vi "Disconnect.vi"(6 "Timeout ms (1000)":i32=1000, 8 "error in (no error)":errorcluster, 11 "NetworkConnection in":refnum<class "NetworkConnection.lvclass">) -> (0 "error out":errorcluster, 3 "NetworkConnection out":refnum<class "NetworkConnection.lvclass">)   [LabVIEW 2020, in "NetworkConnection.lvclass"]
doc: "Disconnects the Network Connection. All unread messages will be flushed.\nJKI Network Streams Connection 1.1.1.15\nJavier Ruiz - JKI\nCopyright (c) 2020, JKI\n\nThis library is provided \"AS IS\" ,WITHOUT WARRANTIES OR CONDITIONS OF ANY KIND, either express or implied."
uses:
  NetworkConnection.lvclass
  Flush And Wait Empty Condition.ctl
  NetworkMessage--Cluster.ctl
  NetworkCommand--Cluster.ctl
  NetworkConnection.lvclass/NetworkConnection.ctl
panel:
  # "Copyright © 2020 JKI All rights reserved.\n\nAuthor: Javier Ruiz <javier.ruiz@jki.net>\n\nThis library is provided \"AS IS\" ,WITHOUT WARRANTIES OR \nCONDITIONS OF ANY KIND, either expressed or implied.\n\nJKI -- jki.net"
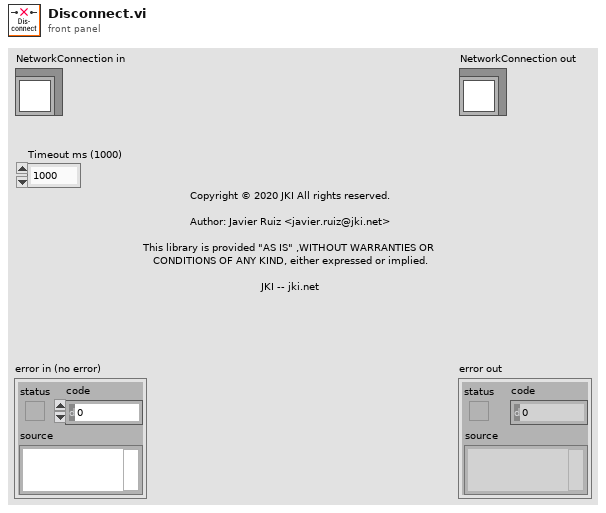
[diagram p1: front panel]
types:
  T1 = typedef "Flush And Wait Empty Condition.ctl" = u8
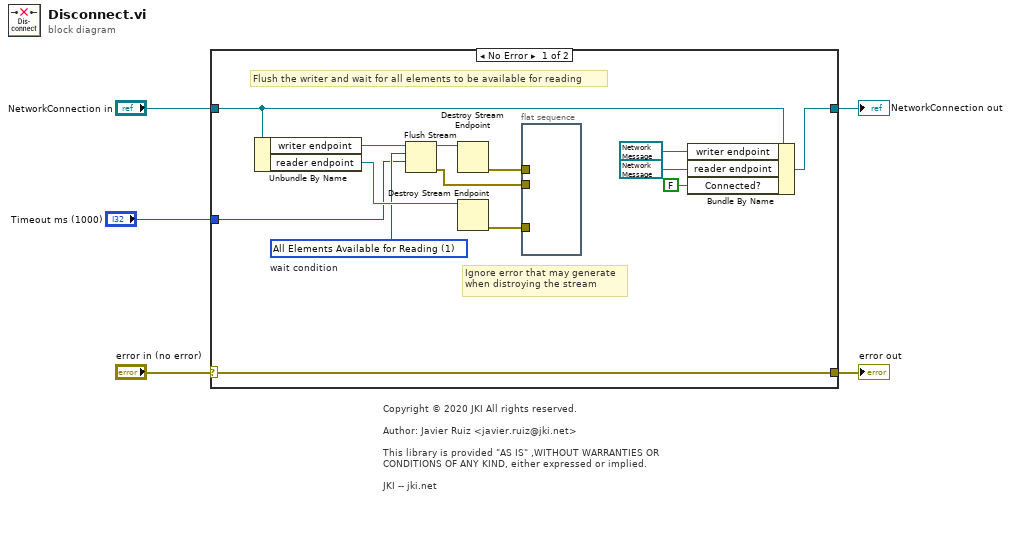
[diagram p0: block diagram]
diagram:
  # "Copyright © 2020 JKI All rights reserved.\n\nAuthor: Javier Ruiz <javier.ruiz@jki.net>\n\nThis library is provided \"AS IS\" ,WITHOUT WARRANTIES OR \nCONDITIONS OF ANY KIND, either expressed or implied.\n\nJKI -- jki.net"
  n1 = case shown="No Error" "error in (no error)" {
    selector: "error in (no error)" -> [w19 w21]
    tunnel: [w19 w21] -> w4
    tunnel: [w16 w20] -> w2
    tunnel: "NetworkConnection in" -> [w17 w20]
    tunnel: "Timeout ms (1000)" -> [w6 _]
    frame No Error {
      w9 = T1 1 items=["All Elements Read From Stream", "All Elements Available for Reading"]  # wait condition
      # "Flush the writer and wait for all elements to be available for reading"
      # "Ignore error that may generate\nwhen distroying the stream"
      n2 = Unbundle By Name(w17) -> ("writer endpoint"=w12:refnum<k21>, "reader endpoint"=w18:refnum<k21>)
      n3 = Flush Stream(9:w6, 10:w9, 11:w12) -> (0:w10:errorcluster, 3:w11:refnum<k21>)  [unwired: 1 in, 1 out]
      n4 = Destroy Stream Endpoint(11:w11) -> (0:w14:errorcluster)  [unwired: 1 in]
      n5 = Destroy Stream Endpoint(11:w18) -> (0:w13:errorcluster)  [unwired: 1 in]
      n6 = flat-sequence {
        tunnel: w14 -> [_]
        tunnel: w13 -> [_]
        tunnel: w10 -> [_]
        frame #0 {
        }
      }
      n7 = Bundle By Name(cluster=w17, "writer endpoint"=refnum<k21> refnum, "reader endpoint"=refnum<k21> refnum, "Connected?"=FALSE) -> (w16:refnum<class "NetworkConnection.lvclass">)
    }
    frame Error {
    }
  }
  "error out" <- w4
  "NetworkConnection out" <- w2
